vi "Control - Generic - Intake Air Desired MAF Host.vi"() -> ()   [LabVIEW 2015, in "ECS-Host.lvlib"]
uses:
  ECS-Host.lvlib
  <vilib>/addons/Software Calibration Management/XControls/TBL2D.xctl
panel:
  in  "MAF_Tbl":cluster{"X":sgl[], "Y":sgl[], "Z":sgl[][]}(xcontrol) caption="[]"
  out "AirMass_Des":sgl caption="[kPa]"
  in  "AirMass_Man":sgl caption="[kPa]"
  in  "AirMass_ManE":bool caption="ManualBoost1SetpointEnable"
  out "VE":sgl caption="[%]"
  out "MAT":sgl caption="[kPa]"
  in  "MAP_ManE":bool caption="ManualBoost1SetpointEnable"
  in  "MAP_Man":sgl caption="[kPa]"
  out "MAP_Des":sgl caption="[kPa]"
  in  "MAP_Max":sgl caption="[kPa]"
  out "MAF_TblOut":sgl caption="[kPa]"
  out "EngineSpeed":sgl caption="[RPM]"
  out "MAP_Calc":sgl caption="[kPa]"
  out "MAP":sgl caption="[kPa]"
  out "MEP_Des":sgl caption="[bar]"
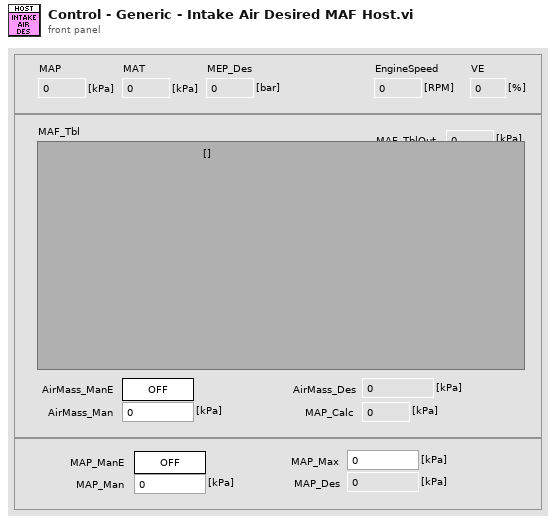
[diagram p1: front panel]
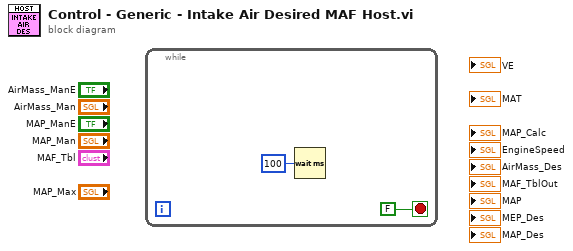
[diagram p0: block diagram]
diagram:
  n1 = while {
    stop <- FALSE stop-if-true
    n2 = Wait (ms)(milliseconds to wait=u32 100) -> ()  [unwired: 1 out]
  }
